vi "close_h264.vi"(8 "error in (no error)":errorcluster, 11 "ir_file_handler":u64) -> (0 "error out":errorcluster, 3 "filename":path)   [LabVIEW 2011, in "librir.lvlib"]
uses:
  librir.lvlib
  libs/video_io.dll
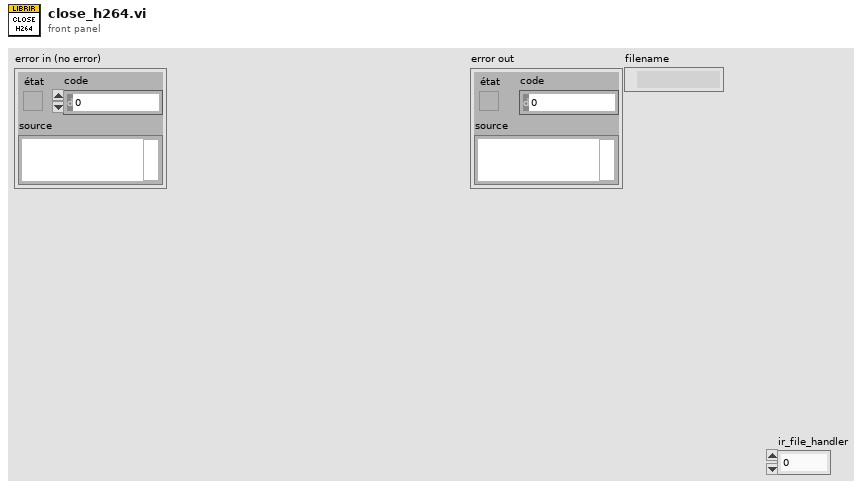
[diagram p1: front panel]
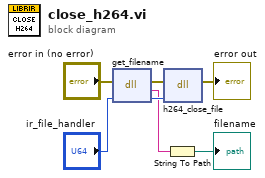
[diagram p0: block diagram]
diagram:
  n1 = dll-call lib="G:/librir/src/labview/libs/video_io.dll" fn="get_filename"(error in="error in (no error)", "ir_file_handler"="ir_file_handler") -> (error out=w3:errorcluster, "filename"=w2:string, "ir_file_handler"=w5:u64)  [unwired: 2 in, 1 out]
  n2 = dll-call lib="G:/librir/src/labview/libs/video_io.dll" fn="h264_close_file"(error in=w3, "ir_file_handler"=w5) -> (error out=→"error out":errorcluster)  [unwired: 4 in, 1 out]
  n3 = String To Path(string=w2) -> (path=→"filename":path)
